vi "Test Executive.vi"(11 "Module Config":T30={"Name"="Test Executive", "Parent Q"=refnum, "Is Child?"=FALSE, "Index"=0, "Dirs"={"Root"=path "C:/MTE", "Config"=path "C:/MTE/Config", "Logs"=path "C:/MTE/Logs", "Reports"=path "C:/ATE/Reports", "App Data"=path "C:/ProgramData/Test Executive"}, "Simulate"=FALSE, "SimCtrl"=refnum}) -> ()   [LabVIEW 2018] (continued)
                          n1454 = control-ref of="Rigth Image"() -> (w3116:refnum<vi>)
                          n1455 = control-ref of="Left Image"() -> (w3115:refnum<vi>)
                          n1456 = call "Image.Load, Zoom and Center.vi"("Zoom Factor"=w3114, "2D Pict Ref"=w3116, "File"=w3125) -> ("error out"=w3117:errorcluster, "2D Pict"=→"Rigth Image":picture)  [unwired: 7 in]
                          n1457 = call "Image.Load, Zoom and Center.vi"("Zoom Factor"=w3114, "2D Pict Ref"=w3115, "File"=w3126) -> ("error out"=w3119:errorcluster, "2D Pict"=→"Left Image":picture)  [unwired: 7 in]
                          n1458 = Merge Errors(w3119, w3117) -> (w3118:errorcluster)
                          n1459 = case shown="Error" w3118 {
                            tunnel: w3122 -> [w3132 w3144]
                            tunnel: [w3132 w3143] -> w3121
                            tunnel: ["Wait for Input" "Result"] -> w3120
                            tunnel: w3117 -> [_ w3137]
                            tunnel: w3119 -> [_ w3138]
                            frame No Error {
                              n1460 = property on="OperNo 2" class="Bool"("DisabledEnum"=T36."Enabled" ("Disabled")) -> (error out=w3129:errorcluster)  [unwired: 2 in, 1 out]
                              n1461 = property on="OperOK 2" class="Bool"(error in=w3129, "DisabledEnum"=T36."Enabled" ("Disabled")) -> (error out=w3127:errorcluster)  [unwired: 1 in, 1 out]
                              n1462 = property on="OperOK 2" class="Bool"(error in=w3127, "Key Focus"=TRUE) -> ()  [unwired: 1 in, 2 out]
                            }
                            frame Error {
                              w3141 = T74 -5200 items=["No Error"=0, "Abort"=-2, "Misc"=-5000, "Fixture Error"=-5100, "File IO - General"=-5200, "FIle IO - Config Error"=-5201, "Instrument - General"=-5300, "Instrument - Serial Com"=-5301, "Instrument - Camera"=-5302, "Instrument - PS"=-5303, "Instrument - Oscilloscope"=-5304, "Instrument - Function Gen"=-5305, "Instrument - Load"=-5306, "Instrument - Meter"=-5307, "Instrument - Power Control"=-5308, "Instrument - Motion"=-5309, "Instrument - RF"=-5310, "System Exe"=-5400, "Image Processing"=-5500, "Communication"=-5600, "Script - Syntax Error"=-6000, "Script - Invalid Name or Param"=-6100, "Script - Timeout"=-6200, "Invalid Data"=-6300, "FW Update Error"=-6500] ("Std Code")
                              w3142 = T39 3 items=["LOG", "PASS", "FAIL", "ERROR"] ("Result.Status")
                              n1463 = case shown="Error" w3138 {
                                tunnel: w3137 -> [w3147 w3150]
                                tunnel: [w3146 w3149] -> w3135
                                frame No Error {
                                n1464 = case shown="Error" w3147 {
                                tunnel: [_ "Right image file load error."] -> w3146
                                frame No Error {
                                # "Will not get here"
                                }
                                frame Error {
                                }
                                }
                                }
                                frame Error {
                                n1465 = case shown="No Error" w3150 {
                                tunnel: ["Left image file load error." "Both left and right image file load error."] -> w3149
                                frame No Error {
                                }
                                frame Error {
                                }
                                }
                                }
                              }
                              n1466 = To Long Integer(number=w3141) -> (32bit integer=w3140:T74)
                              n1467 = Concatenate Strings("Image prompt error.  ", w3135) -> (w3136:string)
                              n1468 = Bundle By Name(cluster=w3144, "Result.Value"="Image Load Error", "Result.Status"=w3142, "Result.Code"=w3140, "Result.Desc"=w3136) -> (w3143:T80)
                            }
                          }
                        }
                        frame "Wait for Input" {
                          n1469 = while {
                            tunnel: w3155 -> [w3158]
                            tunnel: [w3157] -> w3154
                            tunnel: [w3156] -> w3153
                            stop <- w3159 stop-if-true
                            n1470 = event shown="[1] \"OperOK 2\", \"OperNo 2\": Value Change" {
                              selector: _ -> [_ _]
                              dyn-events: _ -> [_ _]
                              timeout: 100 -> [_ _]
                              tunnel: [w3163 TRUE] -> w3159
                              tunnel: w3158 -> [w3162 w3172]
                              tunnel: [w3162 w3171] -> w3157
                              tunnel: ["Done" "Result"] -> w3156
                              event Timeout {
                                n1471 = event-data() -> ()  [unwired: 1 in, 3 out]
                                n1472 = local read "Abort Flag"() -> (w3163:bool)
                              }
                              event "OperOK 2", "OperNo 2": Value Change {
                                n1473 = event-data() -> ()  [unwired: 1 in, 6 out]
                                n1474 = case shown="True" "OperOK 2" {
                                tunnel: ["Reject" "Accept"] -> w3169
                                tunnel: [w3176 w3179] -> w3168
                                tunnel: [5000 _] -> w3167
                                tunnel: ["Operator rejected image" _] -> w3166
                                tunnel: [_ TRUE] -> w3165
                                frame False {
                                w3176 = T39 2 items=["LOG", "PASS", "FAIL", "ERROR"] ("Result.Status")
                                }
                                frame True {
                                w3179 = T39 1 items=["LOG", "PASS", "FAIL", "ERROR"] ("Result.Status")
                                }
                                }
                                n1475 = Bundle By Name(cluster=w3172, "OK"=w3165, "Result.Value"=w3169, "Result.Status"=w3168, "Result.Code"=w3167, "Result.Desc"=w3166) -> (w3171:T80)
                              }
                            }
                          }
                        }
                        frame "Result" {
                          n1476 = Unbundle By Name(w3183) -> ("Result"=w3181:T43)
                          n1477 = Build Array(w3181) -> (w3186:T43[])
                          n1478 = To Variant(anything=w3186) -> (Variant=w3187:variant)
                          n1479 = call <vilib>:"Q.Enqueue Task.vi"("Top of Q"=TRUE, "Data1"=w3187, "Task Name"="Result - Attributes", "Q In"=w3184) -> ()  [unwired: 6 in, 2 out]
                        }
                        frame "Done", Default {
                          n1480 = Unbundle By Name(w3190) -> ("Opts.DispDetails"=w3193:bool)
                          n1481 = Select(t=1, s=w3193, f=0) -> (s? t:f=w3189:i32)
                          n1482 = local write "Test Status Tab"(w3189) -> ()
                          n1483 = local write "Test Status Tab Sel"(w3189) -> ()
                          n1484 = property on="OperNo 2" class="Bool"("DisabledEnum"=T36."Disabled and Grayed Out" ("Disabled")) -> ()  [unwired: 2 in, 2 out]
                          n1485 = property on="OperOK 2" class="Bool"("DisabledEnum"=T36."Disabled and Grayed Out" ("Disabled")) -> ()  [unwired: 2 in, 2 out]
                          n1486 = Unbundle By Name(w3195) -> ("OK"=w3194:bool)
                          n1487 = Select(t="Image Check: PASS" ("Category"), s=w3194, f="Image Check: FAIL" ("Category")) -> (s? t:f=w3200:string)
                          n1488 = property on="Status" class="Str"("Text.Text"=w3200, "Text.BGColor"=u32 13816530, "Blinking"=FALSE) -> ()  [unwired: 2 in, 2 out]
                        }
                      }
                    }
                  }
                  frame "PLCStart" {
                    n1489 = property on="PLC" class="Bool (strict)"() -> ("Visible"=w3206:bool)  [unwired: 2 in, 2 out]
                    n1490 = case shown="True" w3206 {
                      frame False {
                      }
                      frame True {
                        n1491 = call <vilib>:"Q.Enqueue Task.vi"("Q Name"="PLC", "Task Name"="TE PLC Start") -> ()  [unwired: 8 in, 2 out]
                      }
                    }
                  }
                  frame "Print_Label" {
                    # "Print_Label(Print_Text, URL)\n  If 2 arguements then will use this method.\n\nPrint_Label(Print_Text, File,CfgSection,CfgItem)\n  If 2 arguements then will use this method.\n  File can be full path or file name\n  If file name then folder is \"c:\\MTE\\[Test Station]\\Config\\\""
                    n1492 = Index Array(array=w3223) -> (element #1=w3219:string, element #2=w3221:string, element #3=w3220:string, element #4=w3222:string)  [unwired: 4 in]
                    n1493 = Unbundle By Name(w3212) -> ("Cfg.Dirs.Config"=w3211:path)
                    n1494 = Empty String/Path?(string/path=w3220) -> (empty?=w3218:bool)
                    n1495 = case shown="False" w3218 {
                      tunnel: w3222 -> [w3233 _]
                      tunnel: w3221 -> [w3232 w3240]
                      tunnel: w3220 -> [w3234 _]
                      tunnel: w3219 -> [w3235 w3241]
                      tunnel: [_ w3240] -> w3216
                      tunnel: [w3235 w3241] -> w3215
                      tunnel: [w3234 _] -> w3214
                      tunnel: [w3233 _] -> w3213
                      tunnel: w3211 -> [w3228 _]
                      tunnel: [w3225 _] -> w3210
                      frame False {
                        n1496 = String To Path(string=w3232) -> (path=w3226:path)
                        n1497 = Strip Path(path=w3226) -> (stripped path=w3230:path, name=w3227:string)
                        n1498 = Equal?(x=path "" ("stripped path"), y=w3230) -> (x = y?=w3229:bool)
                        n1499 = case shown="True" w3229 {
                          tunnel: w3228 -> [_ w3239]
                          tunnel: w3227 -> [_ w3238]
                          tunnel: w3226 -> [w3236 _]
                          tunnel: [w3236 w3237] -> w3225
                          frame False {
                          }
                          frame True {
                            n1500 = Build Path(base path=w3239, name or relative path=w3238) -> (appended path=w3237:path)
                          }
                        }
                      }
                      frame True {
                        # "Print_Label(URL,Print_Text)"
                      }
                    }
                    n1501 = call "TestExec.Print Label.vi"("CfgItem"=w3213, "URL"=w3216, "CfgSection"=w3214, "Text to Print"=w3215, "Config File"=w3210) -> ("error out"=w3217:errorcluster)  [unwired: 6 in]
                  }
                  frame "ProcessKill" {
                    # "ProcessKill(ProcessName)"
                    n1502 = Index Array(array=w3248) -> (element=w3247:string)  [unwired: 1 in]
                    n1503 = call "CmdExe.Get Processes with Kill Option.vi"("Kill Only 1 Instance"=TRUE, "Name Contains"=FALSE, "Kill Task"=TRUE, "Process Name"=w3247) -> ("Error Out"=w3242:errorcluster)  [unwired: 4 in, 3 out]
                    n1504 = call <vilib>:"Clear Errors.vi"("error in (no error)"=w3242) -> ()  [unwired: 5 in, 2 out]
                  }
                  frame "ProcessStatus" {
                    # "ProcessStatus(ProcessName, [RtnVarName])"
                    n1505 = Index Array(array=w3266) -> (element #1=w3265:string, element #2=w3252:string)  [unwired: 2 in]
                    n1506 = case shown="\"\"" w3252 {
                      selector: w3252 -> [w3267 _]
                      tunnel: [w3267 "ProcessIsRunning"] -> w3251
                      frame Default {
                      }
                      frame "" {
                      }
                    }
                    n1507 = call "CmdExe.Get Processes with Kill Option.vi"("Kill Only 1 Instance"=TRUE, "Name Contains"=FALSE, "Kill Task"=FALSE, "Process Name"=w3265) -> ("Error Out"=w3261:errorcluster, "Is Running"=w3249:bool)  [unwired: 4 in, 2 out]
                    n1508 = call <vilib>:"Clear Errors.vi"("error in (no error)"=w3261) -> ()  [unwired: 5 in, 2 out]
                    n1509 = Select(t="1", s=w3249, f="0") -> (s? t:f=w3254:string)
                    n1510 = Build Array(w3251, w3254) -> (w3253:string[])
                    n1511 = Unbundle By Name(w3257) -> ("SeqMgr"=w3260:refnum<class "SeqMgr.lvclass">)
                    n1512 = Build Array(w3253) -> (w3250:string[][])
                    n1513 = call <vilib>:"SeqMgr.Variables - Add, Replace.vi"("Name, Value"=w3250, "SeqMgr in"=w3260) -> ("SeqMgr out"=w3259:refnum<class "SeqMgr.lvclass">)  [unwired: 8 in, 1 out]
                    n1514 = Bundle By Name(cluster=w3257, "SeqMgr"=w3259) -> (w3258:T73)
                  }
                  frame "ReadINIConfig" {
                    # "ReadINIConfig(Folder,FileName,[Section1,Param1,Section2,Param2,...])\nReturns Vars: ConfigFileExists = 1 if exists, 0 otherwise\nFor each Section/Item pair  Sect1.Param1 = Value1\n                                                 Sect2.Param2 = Value2 . . ."
                    n1515 = while {
                      tunnel: w3270 -> [w3279]
                      shift-right: [w3282] -> w3271
                      shift-left: _ -> [w3283]
                      shift-right: [w3281] -> _
                      shift-left: "Init" -> [w3284]
                      tunnel: w3269 -> [w3278]
                      stop <- w3280 stop-if-true
                      n1516 = case shown="\"Init\"" w3284 {
                        tunnel: w3283 -> [_ w3304 w3314 w3340 w3375]
                        tunnel: [w3288 w3303 w3312 w3341 w3375] -> w3282
                        tunnel: ["File Exists" "Item List" w3313 "Done" _] -> w3281
                        tunnel: [_ _ _ _ TRUE] -> w3280
                        tunnel: w3279 -> [_ w3309 w3311 _ _]
                        tunnel: w3278 -> [_ w3300 _ _ _]
                        tunnel: [_ _ w3310 w3344 _] -> _
                        frame "Init" {
                          w3285 = FALSE  # Exists
                          w3286 = path ""  # Path
                          w3289 = string[][] []  # Items
                          w3290 = string[][] []  # Vars
                          n1517 = Bundle("Vars"=w3290, "Items"=w3289, "Path"=w3286, "Exists"=w3285) -> (w3288:T81)  [unwired: 1 in]
                        }
                        frame "File Exists" {
                          n1518 = Unbundle By Name(w3300) -> ("Cfg.Dirs.Config"=w3298:path)
                          n1519 = Index Array(array=w3309) -> (element #1=w3297:string, element #2=w3294:string)  [unwired: 2 in]
                          n1520 = Empty String/Path?(string/path=w3297) -> (empty?=w3299:bool)
                          n1521 = String To Path(string=w3297) -> (path=w3296:path)
                          n1522 = Select(t=w3298, s=w3299, f=w3296) -> (s? t:f=w3295:path)
                          n1523 = Build Path(base path=w3295, name or relative path=w3294) -> (appended path=w3293:path)
                          n1524 = call <vilib>:"File.Check if File or Folder Exists.vi"("Path"=w3293) -> ("Exists"=w3291:bool)  [unwired: 6 in, 4 out]
                          n1525 = Select(t="1", s=w3291, f="0") -> (s? t:f=w3307:string)
                          n1526 = Build Array("ConfigFileExists", w3307) -> (w3301:string[])
                          n1527 = Build Array(w3301) -> (w3302:string[][])
                          n1528 = Bundle By Name(cluster=w3304, "Path"=w3293, "Vars"=w3302, "Exists"=w3291) -> (w3303:T81)
                        }
                        frame "Item List" {
                          n1529 = Delete From Array(array=w3311, length=2, index=0) -> (array with subset deleted=w3315:string[])  [unwired: 1 out]
                          n1530 = Array Size(array=w3315) -> (size(s)=w3316:i32)
                          n1531 = case shown="Default" w3316 {
                            selector: w3316 -> [_ w3332]
                            tunnel: w3315 -> [_ w3331]
                            tunnel: w3314 -> [w3320 w3327]
                            tunnel: ["Done" "Get Items"] -> w3313
                            tunnel: [w3321 w3326] -> w3312
                            tunnel: [w3319 _] -> w3310
                            frame 0 {
                              n1532 = Unbundle By Name(w3320) -> ("Path"=w3323:path)
                              n1533 = call "File.Config, List Sections and Items in an INI File.vi"("Path"=w3323) -> ("error out"=w3319:errorcluster, "Items"=w3322:string[][])  [unwired: 9 in]
                              n1534 = Bundle By Name(cluster=w3320, "Items"=w3322) -> (w3321:T81)
                            }
                            frame Default {
                              n1535 = To Double Precision Float(number=w3332) -> (double precision float=w3334:dbl)
                              n1536 = Divide(x=w3334, y=2.0) -> (x/y=w3333:dbl)
                              n1537 = To Long Integer(number=w3333) -> (32bit integer=w3330:i32)
                              n1538 = Reshape Array(w3331, w3330, 2 ("dimension size")) -> (w3325:string[][])
                              n1539 = Bundle By Name(cluster=w3327, "Items"=w3325) -> (w3326:T81)
                            }
                          }
                        }
                        frame "Get Items" {
                          n1540 = Unbundle By Name(w3340) -> ("Items"=w3342:string[][], "Path"=w3343:path, "Exists"=w3336:bool)
                          n1541 = case shown="True" w3336 {
                            tunnel: [_ w3362] -> w3344
                            tunnel: w3343 -> [_ w3361]
                            tunnel: w3342 -> [w3347 w3356]
                            tunnel: [w3346 w3355] -> w3337
                            frame False {
                              # "Make empty Vars"
                              n1542 = for {
                                tunnel: w3347 -> [w3354] mode=indexing
                                tunnel: [w3349] -> w3346 mode=indexing
                                n1543 = Index Array(array=w3354) -> (element #1=w3353:string, element #2=w3352:string)  [unwired: 2 in]
                                n1544 = Concatenate Strings(w3353, ".", w3352) -> (w3351:string)
                                n1545 = Build Array(w3351, "") -> (w3349:string[])
                              }
                            }
                            frame True {
                              n1546 = call <vilib>:"Open Config Data.vi"("configuration file path"=w3361) -> ("error out"=w3359:errorcluster, "refnum"=w3360:T82)  [unwired: 8 in, 1 out]
                              n1547 = for {
                                tunnel: w3360 -> [w3374]
                                tunnel: [w3371] -> w3357
                                shift-right: [w3372] -> w3358
                                shift-left: w3359 -> [w3373]
                                tunnel: w3356 -> [w3370] mode=indexing
                                tunnel: [w3364] -> w3355 mode=indexing
                                tunnel: [w3363] -> _
                                n1548 = Index Array(array=w3370) -> (element #1=w3369:string, element #2=w3368:string)  [unwired: 2 in]
                                n1549 = call-poly <vilib>:"Read Key.vi"("section"=w3369, "error in (no error)"=w3373, "key"=w3368, "refnum"=w3374) -> ("error out"=w3372:errorcluster, "value"=w3366:string, "found?"=w3363:bool, "refnum out"=w3371:T82)  [unwired: 4 in]
                                n1550 = Concatenate Strings(w3369, ".", w3368) -> (w3367:string)
                                n1551 = Build Array(w3367, w3366) -> (w3364:string[])
                              }
                              n1552 = call <vilib>:"Close Config Data.vi"("error in (no error)"=w3358, "refnum"=w3357) -> ("error out"=w3362:errorcluster)  [unwired: 8 in, 1 out]
                            }
                          }
                          n1553 = Unbundle By Name(w3340) -> ("Vars"=w3339:string[][])
                          n1554 = Build Array (concatenate)(w3339, w3337) -> (w3338:string[][])
                          n1555 = Bundle By Name(cluster=w3340, "Vars"=w3338) -> (w3341:T81)
                        }
                        frame "Done", Default {
                        }
                      }
                    }
                    n1556 = Unbundle By Name(w3273) -> ("SeqMgr"=w3277:refnum<class "SeqMgr.lvclass">)
                    n1557 = Unbundle By Name(w3271) -> ("Vars"=w3275:string[][])
                    n1558 = call <vilib>:"SeqMgr.Variables - Add, Replace.vi"("Name, Value"=w3275, "SeqMgr in"=w3277) -> ("SeqMgr out"=w3276:refnum<class "SeqMgr.lvclass">)  [unwired: 8 in, 1 out]
                    n1559 = Bundle By Name(cluster=w3273, "SeqMgr"=w3276) -> (w3274:T73)
                  }
                  frame "RepeatMe" {
                    # "RepeatMe(WaitSecs)"
                    n1560 = Index Array(array=w3377) -> (element=w3385:string)  [unwired: 1 in]
                    n1561 = Fract/Exp String To Number(string=w3385) -> (number=w3384:dbl)  [unwired: 3 in, 1 out]
                    n1562 = Bundle By Name(cluster=w3380, "Repeat(s)"=w3384) -> (w3379:T73)
                    n1563 = Greater Or Equal To 0?(x=w3384) -> (x >= 0?=w3383:bool)
                    n1564 = case shown="False" w3383 {
                      tunnel: ["Repeat Sequence turned OFF." w3391] -> w3381
                      tunnel: w3384 -> [_ w3389]
                      frame False {
                      }
                      frame True {
                        n1565 = Number To Fractional String(number=w3389, precision (6)=i16 1) -> (F-format string=w3387:string)  [unwired: 2 in]
                        n1566 = Format Into String(format string="Repeat Sequence turned ON, set for %s secs.", w3387) -> (resulting string=w3391:string)  [unwired: 2 in, 1 out]
                      }
                    }
                    n1567 = Unbundle By Name(w3378) -> ("Log"=w3382:refnum<class "Event Notification.lvclass">)
                    n1568 = call <vilib>:"Event Notification.Status Message.vi"("Message"=w3381, "Event Notification in"=w3382) -> ()  [unwired: 10 in]
                  }
                  frame "RunUtility" {
                    w3393 = TRUE ("Top of Q")
                    n1569 = Index Array(array=w3417) -> (element=w3420:string)  [unwired: 1 in]
                    n1570 = Unbundle By Name(w3416) -> ("Cfg.Dirs.Config"=w3422:path)
                    n1571 = Unbundle By Name(w3394) -> ("UUT Dir"=w3414:path, "TimeOut(s)"=w3415:dbl)
                    n1572 = Unbundle By Name(w3394) -> ("SeqMgr"=w3419:refnum<class "SeqMgr.lvclass">)
                    n1573 = Build Path(base path=w3422, name or relative path=w3420) -> (appended path=w3421:path)
                    n1574 = call <vilib>:"SeqMgr.Variables - Get.vi"("SeqMgr in"=w3419) -> ("Vars"=w3418:variant)  [unwired: 8 in, 2 out]
                    n1575 = call "TestExec.Run Executable and Parse Results V2vi.vi"("Vars"=w3418, "Timeout(s)"=w3415, "Output Folder"=w3414, "Utility Config File"=w3421) -> ("Error"=w3392:errorcluster, "RTN Data"=w3412:T83)  [unwired: 6 in]
                    n1576 = Unbundle By Name(w3412) -> ("Vars"=w3405:string[][], "SW Items"=w3404:T31[], "FileObjs"=w3402:T29[], "MeasData"=w3403:T38[])
                    n1577 = call <vilib>:"Clear Errors.vi"("error in (no error)"=w3392) -> ()  [unwired: 5 in, 2 out]
                    n1578 = To Variant(anything=w3404) -> (Variant=w3397:variant)
                    n1579 = To Variant(anything=w3402) -> (Variant=w3398:variant)
                    n1580 = To Variant(anything=w3403) -> (Variant=w3399:variant)
                    n1581 = call <vilib>:"Q.Enqueue Task.vi"("Top of Q"=w3393, "Data1"=w3399, "Task Name"="Result - Measurements", "Q In"=w3411) -> ("Q Out"=w3400:refnum<queue>)  [unwired: 6 in, 1 out]
                    n1582 = local read "Variables"() -> (w3409:string[][])
                    n1583 = Unbundle By Name(w3394) -> ("SeqMgr"=w3407:refnum<class "SeqMgr.lvclass">)
                    n1584 = call <vilib>:"Q.Enqueue Task.vi"("Top of Q"=w3393, "Data1"=w3398, "Task Name"="Result - File Objs" ("Cmd"), "Q In"=w3400) -> ("Q Out"=w3401:refnum<queue>)  [unwired: 6 in, 1 out]
                    n1585 = call <vilib>:"Q.Enqueue Task.vi"("Top of Q"=w3393, "Data1"=w3397, "Task Name"="Client - SW Items", "Q In"=w3401) -> ()  [unwired: 6 in, 2 out]
                    n1586 = call "TestExec.Add New 1D Items to 2D List, Overwrite if is existing.vi"("New Items"=w3405, "Item List"=w3409) -> ("Item List Out"=w3410:string[][])  [unwired: 9 in]
                    n1587 = call <vilib>:"SeqMgr.Variables - Add, Replace.vi"("Name, Value"=w3405, "SeqMgr in"=w3407) -> ("SeqMgr out"=w3408:refnum<class "SeqMgr.lvclass">)  [unwired: 8 in, 1 out]
                    n1588 = Bundle By Name(cluster=w3394, "SeqMgr"=w3408) -> (w3406:T73)
                    n1589 = local write "Variables"(w3410) -> ()
                  }
                  frame "RunExe" {
                    n1590 = Unbundle By Name(w3435) -> ("UUT Dir"=w3430:path, "TimeOut(s)"=w3439:dbl)
                    n1591 = Delete From Array(array=w3429, length=1, index=0) -> (deleted portion=w3423:string[], array with subset deleted=w3425:string[])
                    n1592 = Unbundle By Name(w3435) -> ("SeqMgr"=w3441:refnum<class "SeqMgr.lvclass">)
                    n1593 = Index Array(array=w3423) -> (element=w3424:string)  [unwired: 1 in]
                    n1594 = local write "Args"(w3425) -> ()
                    n1595 = call <vilib>:"SeqMgr.Variables - Get.vi"("SeqMgr in"=w3441) -> ("Vars"=w3440:variant)  [unwired: 8 in, 2 out]
                    n1596 = String To Path(string=w3424) -> (path=w3426:path)
                    n1597 = local write "Exe Path"(w3426) -> ()
                    n1598 = call "TestExec.Run Executable and Rtn.vi"("Vars"=w3440, "Timeout(s)"=w3439, "Log Dir"=w3430, "Input"=w3429) -> ("Error"=w3431:errorcluster, "RTN Data"=w3434:T83)  [unwired: 6 in]
                    n1599 = call <vilib>:"Clear Errors.vi"("error in (no error)"=w3431) -> ()  [unwired: 5 in, 2 out]
                    n1600 = Unbundle By Name(w3434) -> ("MeasData"=w3433:T38[])
                    n1601 = To Variant(anything=w3433) -> (Variant=w3436:variant)
                    n1602 = call <vilib>:"Q.Enqueue Task.vi"("Top of Q"=TRUE, "Data1"=w3436, "Task Name"="Result - Measurements", "Q In"=w3437) -> ()  [unwired: 6 in, 2 out]
                  }
                  frame "SectionStart" {
                    # "SectionStart(Name)"
                    n1603 = Unbundle By Name(w3446) -> ("SectCtr"=w3466:T72, "Data.Meas"=w3463:T38[])
                    n1604 = Index Array(array=w3442) -> (element=w3459:string)  [unwired: 1 in]
                    n1605 = To Upper Case(1:w3459) -> (0:w3452:string)
                    n1606 = call <vilib>:"Q.Enqueue Task.vi"("Top of Q"=TRUE, "Task Name"="Update Result Table", "Q In"=w3443) -> ()  [unwired: 7 in, 2 out]
                    n1607 = call "Step Counter.Step Count Controller.vi"("Step Action"=Step_Counter.Action."Section Start", "Step State"=w3466) -> ("Step"=w3461:string, "Step State Out"=w3465:T72, "Cntr"=w3454:i32)  [unwired: 7 in]
                    n1608 = Bundle By Name(cluster=T38 {"Cnt"=0, "Step"="", "Category"="", "Name"="", "Value"="", "Units"="", "LimType"="", "LL"="", "UL"="", "Status"=0, "Code"=0, "Desc"="", "Time"=timestamp(0 s since 1904-01-01)} ("Meas"), "Step"=w3461, "Cnt"=w3454, "Category"="Heading", "Name"=w3452, "Value"="==================") -> (w3458:T38)
                    n1609 = Build Array (concatenate)(w3463, w3458) -> (w3462:T38[])
                    n1610 = Bundle By Name(cluster=w3446, "SectCtr"=w3465, "Data.Meas"=w3462) -> (w3445:T73)
                    n1611 = Unbundle By Name(w3444) -> ("Log"=w3451:refnum<class "Event Notification.lvclass">)
                    n1612 = Format Into String(format string="Section Start: %s", w3452) -> (resulting string=w3450:string)  [unwired: 2 in, 1 out]
                    n1613 = call <vilib>:"Event Notification.Status Message.vi"("Log"=TRUE, "Level"=Event_Log.Log_Level."Verbose", "Message"=w3450, "Event Notification in"=w3451) -> ()  [unwired: 8 in]
                  }
                  frame "SendDataToSta" {
                    n1614 = Unbundle By Name(w3469) -> ("ResultState"=w3473:T63, "Data.Meas"=w3468:T38[], "StaApp"=w3467:string)
                    n1615 = To Variant(anything=w3468) -> (Variant=w3470:variant)
                    n1616 = call <vilib>:"Q.Enqueue Task.vi"("Top of Q"=TRUE, "Data1"=w3470, "Q Name"=w3467, "Task Name"="Test Meas Data") -> ()  [unwired: 6 in, 2 out]
                    n1617 = To Variant(anything=w3473) -> (Variant=w3474:variant)
                    n1618 = call <vilib>:"Q.Enqueue Task.vi"("Top of Q"=TRUE, "Data1"=w3474, "Q Name"=w3467, "Task Name"="Test Status") -> ()  [unwired: 6 in, 2 out]
                  }
                  frame "SequenceConfig" {
                    # "If name exists, over write.\nElse append."
                    # "SequenceConfig(Name, Value)"
                    n1619 = Unbundle By Name(w3479) -> ("RptHdr.Test Sequence"=w3489:T49)
                    n1620 = Unbundle By Name(w3489) -> ("Config.Config_Item"=w3486:cluster{"Name":string, "Value":string}[])
                    n1621 = for {
                      tunnel: w3486 -> [w3498] mode=indexing
                      tunnel: [w3497] -> w3485 mode=indexing
                      n1622 = Unbundle By Name(w3498) -> ("Name"=w3497:string)
                    }
                    n1623 = Index Array(array=w3477) -> (element #1=w3480:string, element #2=w3483:string)  [unwired: 2 in]
                    n1624 = Bundle By Name(cluster=cluster{"Name":string, "Value":string} {"Name"="", "Value"=""} ("Setup"), "Name"=w3480, "Value"=w3483) -> (w3482:cluster{"Name":string, "Value":string})
                    n1625 = Search 1D Array(1D array=w3485, element=w3480) -> (index of element=w3481:i32)  [unwired: 1 in]
                    n1626 = case shown="0, Default" w3481 {
                      selector: w3481 -> [w3490 _]
                      tunnel: w3486 -> [w3493 w3496]
                      tunnel: [w3492 w3495] -> w3488
                      tunnel: w3482 -> [w3491 w3494]
                      frame 0, Default {
                        n1627 = Replace Array Subset(array=w3493, new element=w3491, index=w3490) -> (w3492:cluster{"Name":string, "Value":string}[])
                      }
                      frame -1 {
                        n1628 = Build Array (concatenate)(w3496, w3494) -> (w3495:cluster{"Name":string, "Value":string}[])
                      }
                    }
                    n1629 = Bundle By Name(cluster=w3489, "Config.Config_Item"=w3488) -> (w3487:T49)
                    n1630 = Bundle By Name(cluster=w3479, "RptHdr.Test Sequence"=w3487) -> (w3478:T73)
                  }
                  frame "SetDisableResults" {
                    # "SetDisableResults(Enabled)\n1 = Enabled, 0 = Disabled"
                    n1631 = Index Array(array=w3499) -> (element=w3512:string)  [unwired: 1 in]
                    n1632 = Unbundle By Name(w3500) -> ("Opts.DisResults"=w3507:bool)
                    n1633 = Equal?(x=w3512, y="1") -> (x = y?=w3509:bool)
                    n1634 = Or(x=w3507, y=w3509) -> (x .or. y?=w3508:bool)
                    n1635 = Select(t="ON", s=w3509, f="OFF") -> (s? t:f=w3510:string)
                    n1636 = Bundle By Name(cluster=w3500, "DisableResults"=w3508) -> (w3502:T73)
                    n1637 = Unbundle By Name(w3501) -> ("Log"=w3506:refnum<class "Event Notification.lvclass">)
                    n1638 = Format Into String(format string="Set Disable Results to %s.", w3510) -> (resulting string=w3505:string)  [unwired: 2 in, 1 out]
                    n1639 = call <vilib>:"Event Notification.Status Message.vi"("Log"=TRUE, "Level"=Event_Log.Log_Level."Verbose", "Message"=w3505, "Event Notification in"=w3506) -> ()  [unwired: 8 in]
                  }
                  frame "SetSN" {
                    n1640 = Index Array(array=w3535) -> (element=w3525:string)  [unwired: 1 in]
                    n1641 = Unbundle By Name(w3522) -> ("Opts.SNRouteCk"=w3521:bool, "Opts.NotValSN"=w3527:bool, "Lists.UUTRoutes"=w3520:string[])
                    n1642 = Unbundle By Name(w3522) -> ("StaApp"=w3533:string)
                    n1643 = Bundle By Name(cluster=w3522, "RptUUT.UUTInfo.SN"=w3525) -> (w3518:T73)
                    n1644 = To Variant(anything=w3525) -> (Variant=w3531:variant)
                    n1645 = local write "SN"(w3525) -> ()
                    n1646 = local write "SN Rslt"(w3525) -> ()
                    n1647 = call <vilib>:"Q.Enqueue Task.vi"("Data1"=w3531, "Q Name"=w3533, "Task Name"="Update SN") -> ()  [unwired: 7 in, 2 out]
                    n1648 = Format Into String(format string="Sequence reassigned SN to %s" ("Message"), w3525) -> (resulting string=w3538:string)  [unwired: 2 in, 1 out]
                    n1649 = Build Array("SN", w3525) -> (w3524:string[])
                    n1650 = Unbundle By Name(w3526) -> ("Log"=w3539:refnum<class "Event Notification.lvclass">)
                    n1651 = Build Array(w3524) -> (w3523:string[][])
                    n1652 = case shown="True" w3527 {
                      tunnel: [w3550 _] -> _
                      tunnel: w3525 -> [w3549 _]
                      tunnel: w3523 -> [w3548 w3566]
                      tunnel: [w3546 w3566] -> w3516
                      tunnel: [w3543 w3565] -> w3517
                      tunnel: w3521 -> [w3542 _]
                      tunnel: w3520 -> [w3541 _]
                      tunnel: w3518 -> [w3540 w3565]
                      frame False {
                        n1653 = control-ref of="SN"() -> (w3551:refnum<vi>)
                        n1654 = call "TestExec.SN Valid and Route Check.vi"("Process Steps"=w3541, "SN Indicator"=w3551, "SN"=w3549, "Route Check"=w3542) -> ("Message"=w3544:string, "Status"=w3545:bool, "error IO"=w3550:errorcluster)  [unwired: 4 in, 1 out]
                        n1655 = case shown="True" w3545 {
                          tunnel: w3548 -> [w3560 w3564]
                          tunnel: string[][] [["Error", "1"]] ("appended array") -> [w3559 _]
                          tunnel: [w3558 w3564] -> w3546
                          tunnel: w3540 -> [w3555 w3562]
                          tunnel: [w3556 w3561] -> w3543
                          tunnel: w3544 -> [w3553 _]
                          frame False {
                            n1656 = Build Array (concatenate)(w3560, w3559) -> (w3558:string[][])
                            n1657 = local write "UUT SN Status"(w3553) -> ()
                            n1658 = Bundle By Name(cluster=w3555, "PreTestCk.SNErr"=TRUE, "ResultState.State"=SeqMgr.Result_State_Enum."ERROR" ("State"), "ResultState.Code"=-8002, "ResultState.Description"=w3553) -> (w3556:T73)
                          }
                          frame True {
                            # "SN is OK"
                            n1659 = Bundle By Name(cluster=w3562, "PreTestCk.SNErr"=FALSE) -> (w3561:T73)
                          }
                        }
                      }
                      frame True {
                      }
                    }
                    n1660 = call <vilib>:"Event Notification.Status Message.vi"("Display"=TRUE ("Log"), "Level"=Event_Log.Log_Level."Verbose", "Message"=w3538, "Event Notification in"=w3539) -> ()  [unwired: 8 in]
                    n1661 = Unbundle By Name(w3517) -> ("SeqMgr"=w3530:refnum<class "SeqMgr.lvclass">)
                    n1662 = call <vilib>:"SeqMgr.Variables - Add, Replace.vi"("Name, Value"=w3516, "SeqMgr in"=w3530) -> ("SeqMgr out"=w3529:refnum<class "SeqMgr.lvclass">)  [unwired: 8 in, 1 out]
                    n1663 = Bundle By Name(cluster=w3517, "SeqMgr"=w3529) -> (w3519:T73)
                  }
                  frame "SetTimeout" {
                    n1664 = Index Array(array=w3570) -> (element=w3581:string)  [unwired: 1 in]
                    n1665 = Fract/Exp String To Number(string=w3581) -> (number=w3580:dbl)  [unwired: 3 in, 1 out]
                    n1666 = In Range and Coerce(upper limit=1000.0, x=w3580, lower limit=1.0) -> (coerced(x)=w3578:dbl)  [unwired: 1 out]
                    n1667 = call <vilib>:"Q.Enqueue Task.vi"("Top of Q"=TRUE, "Task Name"="Sta Set TimeOut", "Q In"=w3568) -> ()  [unwired: 7 in, 2 out]
                    n1668 = Bundle By Name(cluster=w3572, "TimeOut(s)"=w3578) -> (w3571:T73)
                    n1669 = Unbundle By Name(w3573) -> ("Log"=w3577:refnum<class "Event Notification.lvclass">)
                    n1670 = Format Into String(format string="Function call timeout set to %.2f secs.", w3578) -> (resulting string=w3576:string)  [unwired: 2 in, 1 out]
                    n1671 = call <vilib>:"Event Notification.Status Message.vi"("Log"=TRUE, "Level"=Event_Log.Log_Level."Verbose", "Message"=w3576, "Event Notification in"=w3577) -> ()  [unwired: 8 in]
                  }
                  frame "GetTimeSecs" {
                    n1672 = Index Array(array=w3588) -> (element=w3585:string)  [unwired: 1 in]
                    n1673 = call <vilib>:"High Resolution Relative Seconds.vi"() -> ("relative seconds"=w3587:dbl)
                    n1674 = Number To Fractional String(number=w3587) -> (F-format string=w3586:string)  [unwired: 3 in]
                    n1675 = Build Array(w3585, w3586) -> (w3584:string[])
                    n1676 = Unbundle By Name(w3590) -> ("SeqMgr"=w3593:refnum<class "SeqMgr.lvclass">)
                    n1677 = Build Array(w3584) -> (w3591:string[][])
                    n1678 = call <vilib>:"SeqMgr.Variables - Add, Replace.vi"("Name, Value"=w3591, "SeqMgr in"=w3593) -> ("SeqMgr out"=w3592:refnum<class "SeqMgr.lvclass">)  [unwired: 8 in, 1 out]
                    n1679 = Bundle By Name(cluster=w3590, "SeqMgr"=w3592) -> (w3589:T73)
                  }
                  frame "GetDurationSecs" {
                    n1680 = Index Array(array=w3601) -> (element #1=w3599:string, element #2=w3597:string)  [unwired: 2 in]
                    n1681 = Fract/Exp String To Number(string=w3597) -> (number=w3595:dbl)  [unwired: 3 in, 1 out]
                    n1682 = call <vilib>:"High Resolution Relative Seconds.vi"() -> ("relative seconds"=w3596:dbl)
                    n1683 = Subtract(x=w3596, y=w3595) -> (x-y=w3594:dbl)
                    n1684 = Number To Fractional String(number=w3594) -> (F-format string=w3600:string)  [unwired: 3 in]
                    n1685 = Build Array(w3599, w3600) -> (w3598:string[])
                    n1686 = Unbundle By Name(w3603) -> ("SeqMgr"=w3606:refnum<class "SeqMgr.lvclass">)
                    n1687 = Build Array(w3598) -> (w3604:string[][])
                    n1688 = call <vilib>:"SeqMgr.Variables - Add, Replace.vi"("Name, Value"=w3604, "SeqMgr in"=w3606) -> ("SeqMgr out"=w3605:refnum<class "SeqMgr.lvclass">)  [unwired: 8 in, 1 out]
                    n1689 = Bundle By Name(cluster=w3603, "SeqMgr"=w3605) -> (w3602:T73)
                  }
                  frame "SetVar", "SetVariable" {
                    # "SetVariable(Name,Value)"
                    n1690 = Unbundle By Name(w3609) -> ("SeqMgr"=w3620:refnum<class "SeqMgr.lvclass">)
                    n1691 = Index Array(array=w3607) -> (element #1=w3616:string, element #2=w3615:string)  [unwired: 2 in]
                    n1692 = Build Array(w3607) -> (w3618:string[][])
                    n1693 = call <vilib>:"SeqMgr.Variables - Add, Replace.vi"("Name, Value"=w3618, "SeqMgr in"=w3620) -> ("SeqMgr out"=w3619:refnum<class "SeqMgr.lvclass">)  [unwired: 8 in, 1 out]
                    n1694 = Bundle By Name(cluster=w3609, "SeqMgr"=w3619) -> (w3608:T73)
                    n1695 = Format Into String(format string="Set Var, %s, %s", w3616, w3615) -> (resulting string=w3613:string)  [unwired: 2 in, 1 out]
                    n1696 = Unbundle By Name(w3610) -> ("Log"=w3614:refnum<class "Event Notification.lvclass">)
                    n1697 = call <vilib>:"Event Notification.Status Message.vi"("Log"=TRUE, "Level"=Event_Log.Log_Level."Debug0", "Message"=w3613, "Event Notification in"=w3614) -> ()  [unwired: 8 in]
                  }
                  frame "SubSectionEnd" {
                    # "SubSectionEnd()"
                    n1698 = Unbundle By Name(w3622) -> ("SectCtr"=w3625:T72)
                    n1699 = call "Step Counter.Step Count Controller.vi"("Step Action"=Step_Counter.Action."Sub Section End", "Step State"=w3625) -> ("Step State Out"=w3624:T72)  [unwired: 7 in, 2 out]
                    n1700 = Bundle By Name(cluster=w3622, "SectCtr"=w3624) -> (w3621:T73)
                  }
                  frame "SubSectionStart" {
                    # "SubSectionStart(Name)"
                    n1701 = Index Array(array=w3629) -> (element=w3642:string)  [unwired: 1 in]
                    n1702 = To Upper Case(1:w3642) -> (0:w3639:string)
                    n1703 = Unbundle By Name(w3628) -> ("SectCtr"=w3647:T72, "Data.Meas"=w3645:T38[])
                    n1704 = call <vilib>:"Q.Enqueue Task.vi"("Top of Q"=TRUE, "Task Name"="Update Result Table", "Q In"=w3648) -> ()  [unwired: 7 in, 2 out]
                    n1705 = call "Step Counter.Step Count Controller.vi"("Step Action"=Step_Counter.Action."Sub Section Start", "Step State"=w3647) -> ("Step"=w3643:string, "Step State Out"=w3646:T72, "Cntr"=w3640:i32)  [unwired: 7 in]
                    n1706 = Bundle By Name(cluster=T38 {"Cnt"=0, "Step"="", "Category"="", "Name"="", "Value"="", "Units"="", "LimType"="", "LL"="", "UL"="", "Status"=0, "Code"=0, "Desc"="", "Time"=timestamp(0 s since 1904-01-01)} ("Meas"), "Step"=w3643, "Cnt"=w3640, "Category"="Heading", "Name"=w3639, "Value"="- - - - - - - - - -" ("Category")) -> (w3641:T38)
                    n1707 = Build Array (concatenate)(w3645, w3641) -> (w3644:T38[])
                    n1708 = Bundle By Name(cluster=w3628, "SectCtr"=w3646, "Data.Meas"=w3644) -> (w3626:T73)
                    n1709 = Unbundle By Name(w3627) -> ("Log"=w3638:refnum<class "Event Notification.lvclass">)
                    n1710 = Format Into String(format string="SubSection Start: %s", w3639) -> (resulting string=w3637:string)  [unwired: 2 in, 1 out]
                    n1711 = call <vilib>:"Event Notification.Status Message.vi"("Log"=TRUE, "Level"=Event_Log.Log_Level."Verbose", "Message"=w3637, "Event Notification in"=w3638) -> ()  [unwired: 8 in]
                  }
                  frame "TimeLog" {
                    n1712 = Index Array(array=w3652) -> (element=w3655:string)  [unwired: 1 in]
                    n1713 = Unbundle By Name(w3653) -> ("Log"=w3656:refnum<class "Event Notification.lvclass">)
                    n1714 = call <vilib>:"Event Notification.Status Message.vi"("Display"=TRUE, "Log"=TRUE, "Level"=Event_Log.Log_Level."Normal", "Message"=w3655, "Event Notification in"=w3656) -> ()  [unwired: 7 in]
                  }
                  frame "XlinkPartInitReport" {
                    # "XlinkPartInitReport(DestinationFolder,Batch,Name)"
                    n1715 = Unbundle By Name(w3660) -> ("RptHdr.Test Run.Start Time"=w3668:timestamp, "RptUUT.UUTInfo.SN"=w3667:string, "RptHdr.Test Run.Operator"=w3666:string)
                    n1716 = Index Array(array=w3659) -> (element #1=w3663:string, element #2=w3662:string, element #3=w3661:string)  [unwired: 3 in]
                    n1717 = String To Path(string=w3663) -> (path=w3664:path)
                    n1718 = call "Result.Generate Xlink PN Init Report XML.vi"("Name"=w3661, "Batch"=w3662, "Time Offset"=-1.0, "Folder"=w3664, "Operator"=w3666, "SN"=w3667, "StartTime"=w3668) -> ()  [unwired: 3 in, 2 out]
                  }
                  frame Default {
                    w3672 = T74 -6100 items=["No Error"=0, "Abort"=-2, "Misc"=-5000, "Fixture Error"=-5100, "File IO - General"=-5200, "FIle IO - Config Error"=-5201, "Instrument - General"=-5300, "Instrument - Serial Com"=-5301, "Instrument - Camera"=-5302, "Instrument - PS"=-5303, "Instrument - Oscilloscope"=-5304, "Instrument - Function Gen"=-5305, "Instrument - Load"=-5306, "Instrument - Meter"=-5307, "Instrument - Power Control"=-5308, "Instrument - Motion"=-5309, "Instrument - RF"=-5310, "System Exe"=-5400, "Image Processing"=-5500, "Communication"=-5600, "Script - Syntax Error"=-6000, "Script - Invalid Name or Param"=-6100, "Script - Timeout"=-6200, "Invalid Data"=-6300, "FW Update Error"=-6500] ("Std Code")
                    n1719 = Format Into String(format string="Invalid sequence function name: \"%s\".", w3670) -> (resulting string=w3673:string)  [unwired: 2 in, 1 out]
                    n1720 = call "Error.Set-Change Error Info.vi"("Std Code"=w3672, "Description"=w3673, "Set Error"=TRUE) -> ("error out"=w3669:errorcluster)  [unwired: 8 in]
                  }
                }
              }
              frame Error {
                w3681 = T74 -6000 items=["No Error"=0, "Abort"=-2, "Misc"=-5000, "Fixture Error"=-5100, "File IO - General"=-5200, "FIle IO - Config Error"=-5201, "Instrument - General"=-5300, "Instrument - Serial Com"=-5301, "Instrument - Camera"=-5302, "Instrument - PS"=-5303, "Instrument - Oscilloscope"=-5304, "Instrument - Function Gen"=-5305, "Instrument - Load"=-5306, "Instrument - Meter"=-5307, "Instrument - Power Control"=-5308, "Instrument - Motion"=-5309, "Instrument - RF"=-5310, "System Exe"=-5400, "Image Processing"=-5500, "Communication"=-5600, "Script - Syntax Error"=-6000, "Script - Invalid Name or Param"=-6100, "Script - Timeout"=-6200, "Invalid Data"=-6300, "FW Update Error"=-6500] ("Std Code")
                n1721 = call <vilib>:"Space Constant.vi"() -> ("String"=w3678:string)
                n1722 = Concatenate Strings(w3680, w3678, w3679) -> (w3677:string)
                n1723 = Format Into String(format string="Invalid Data to task %s. Expected 1D string.", w3677) -> (resulting string=w3682:string)  [unwired: 2 in, 1 out]
                n1724 = call "Error.Set-Change Error Info.vi"("Std Code"=w3681, "Description"=w3682) -> ("error out"=w3676:errorcluster)  [unwired: 9 in]
              }
            }
          }
          frame "Set Comment" {
            # "Set SN(SN)"
            n1725 = Variant To Data(type="", Variant=w3697) -> (data=w3686:string)  [unwired: 1 in, 1 out]
            n1726 = Bundle By Name(cluster=w3696, "RptHdr.Test Run.Comment"=w3686) -> (w3693:T73)
            n1727 = local write "Comment"(w3686) -> ()
            n1728 = String Length(string=w3686) -> (length=w3687:i32)
            n1729 = case shown="0..18" w3687 {
              tunnel: [u32 16 ("F2") u32 20 ("F1")] -> w3685
              frame Default {
              }
              frame 0..18 {
              }
            }
            n1730 = Format Into String(format string="Automation reassigned Comment to %s" ("Message"), w3686) -> (resulting string=w3688:string)  [unwired: 2 in, 1 out]
            n1731 = Unbundle By Name(w3689) -> ("Log"=w3692:refnum<class "Event Notification.lvclass">)
            n1732 = property on="SN" class="Str"("Text.FontSize"=w3685) -> ()  [unwired: 2 in, 2 out]
            n1733 = call <vilib>:"Event Notification.Status Message.vi"("Log"=TRUE, "Level"=Event_Log.Log_Level."Verbose", "Message"=w3688, "Event Notification in"=w3692) -> ()  [unwired: 8 in]
          }
          frame "Set Sequence" {
            # "Set Position(Int)"
            n1734 = Variant To Data(type="", Variant=w3714) -> (data=w3701:string)  [unwired: 1 in, 1 out]
            n1735 = property on="Sequence" class="Ring (strict)"() -> ("Strings []"=w3706:string[])  [unwired: 2 in, 2 out]
            n1736 = To Lower Case(string=w3701) -> (all lower case string=w3704:string)
            n1737 = To Lower Case(string=w3706) -> (all lower case string=w3705:string[])
            n1738 = Search 1D Array(1D array=w3705, element=w3704) -> (index of element=w3702:i32)  [unwired: 1 in]
            n1739 = case shown="0, Default" w3702 {
              selector: w3702 -> [_ w3721]
              tunnel: w3701 -> [w3716 _]
              tunnel: [w3715 _] -> w3700
              frame -1 {
                w3719 = T74 -6100 items=["No Error"=0, "Abort"=-2, "Misc"=-5000, "Fixture Error"=-5100, "File IO - General"=-5200, "FIle IO - Config Error"=-5201, "Instrument - General"=-5300, "Instrument - Serial Com"=-5301, "Instrument - Camera"=-5302, "Instrument - PS"=-5303, "Instrument - Oscilloscope"=-5304, "Instrument - Function Gen"=-5305, "Instrument - Load"=-5306, "Instrument - Meter"=-5307, "Instrument - Power Control"=-5308, "Instrument - Motion"=-5309, "Instrument - RF"=-5310, "System Exe"=-5400, "Image Processing"=-5500, "Communication"=-5600, "Script - Syntax Error"=-6000, "Script - Invalid Name or Param"=-6100, "Script - Timeout"=-6200, "Invalid Data"=-6300] ("Std Code")
                n1740 = Format Into String(format string="Error attempted to set to nonexistant sequence: \"%s\"." ("Description"), w3716) -> (resulting string=w3717:string)  [unwired: 2 in, 1 out]
                n1741 = call "Error.Set-Change Error Info.vi"("Std Code"=w3719, "Description"=w3717, "Set Error"=TRUE) -> ("error out"=w3715:errorcluster)  [unwired: 8 in]
              }
              frame 0, Default {
                n1742 = To Unsigned Word Integer(number=w3721) -> (unsigned 16bit integer=w3722:u16)
                n1743 = property on="Sequence" class="Ring (strict)"("Value"=w3722) -> ()  [unwired: 2 in, 2 out]
              }
            }
            n1744 = Unbundle By Name(w3711) -> ("Log"=w3710:refnum<class "Event Notification.lvclass">)
            n1745 = Format Into String(format string="Set Sequence to %s" ("Message"), w3701) -> (resulting string=w3703:string)  [unwired: 2 in, 1 out]
            n1746 = call <vilib>:"Event Notification.Status Message.vi"("Log"=TRUE, "Level"=Event_Log.Log_Level."Normal", "Message"=w3703, "Event Notification in"=w3710) -> ()  [unwired: 8 in]
          }
          frame "Set SN" {
            # "Set SN(SN)"
            n1747 = Variant To Data(type="", Variant=w3739) -> (data=w3725:string)  [unwired: 1 in, 1 out]
            n1748 = Bundle By Name(cluster=w3738, "RptUUT.UUTInfo.SN"=w3725) -> (w3724:T73)
            n1749 = local write "SN"(w3725) -> ()
            n1750 = local write "SN Rslt"(w3725) -> ()
            n1751 = Build Array("SN", w3725) -> (w3726:string[])
            n1752 = Unbundle By Name(w3724) -> ("SeqMgr"=w3730:refnum<class "SeqMgr.lvclass">)
            n1753 = Build Array(w3726) -> (w3728:string[][])
            n1754 = call <vilib>:"SeqMgr.Variables - Add, Replace.vi"("Name, Value"=w3728, "SeqMgr in"=w3730) -> ("SeqMgr out"=w3729:refnum<class "SeqMgr.lvclass">)  [unwired: 8 in, 1 out]
            n1755 = Bundle By Name(cluster=w3724, "SeqMgr"=w3729) -> (w3723:T73)
            n1756 = Format Into String(format string="Automation reassigned SN to %s" ("Message"), w3725) -> (resulting string=w3731:string)  [unwired: 2 in, 1 out]
            n1757 = Unbundle By Name(w3732) -> ("Log"=w3735:refnum<class "Event Notification.lvclass">)
            n1758 = call <vilib>:"Event Notification.Status Message.vi"("Log"=TRUE, "Level"=Event_Log.Log_Level."Verbose", "Message"=w3731, "Event Notification in"=w3735) -> ()  [unwired: 8 in]
          }
          frame "Set UUT Pos" {
            # "Set Position(Int)"
            n1759 = Variant To Data(type="", Variant=w3751) -> (data=w3741:string)  [unwired: 1 in, 1 out]
            n1760 = local write "Position"(w3741) -> ()
            n1761 = property on="Position" class="Str"("Visible"=TRUE) -> ()  [unwired: 2 in, 2 out]
            n1762 = Bundle By Name(cluster=w3750, "RptUUT.Position"=w3741) -> (w3747:T73)
            n1763 = Unbundle By Name(w3746) -> ("Log"=w3744:refnum<class "Event Notification.lvclass">)
            n1764 = Format Into String(format string="UUT Position is %s" ("Message"), w3741) -> (resulting string=w3745:string)  [unwired: 2 in, 1 out]
            n1765 = call <vilib>:"Event Notification.Status Message.vi"("Log"=TRUE, "Level"=Event_Log.Log_Level."Verbose", "Message"=w3745, "Event Notification in"=w3744) -> ()  [unwired: 8 in]
          }
          frame "Set Variables" {
            # "SetVariable(Name,Value)"
            n1766 = Variant To Data(type=string[][] [], Variant=w3765) -> (data=w3753:string[][], error out=w3759:errorcluster)  [unwired: 1 in]
            n1767 = Unbundle By Name(w3763) -> ("SeqMgr"=w3762:refnum<class "SeqMgr.lvclass">)
            n1768 = local read "Variables"() -> (w3754:string[][])
            n1769 = call <vilib>:"SeqMgr.Variables - Add, Replace.vi"("Name, Value"=w3753, "SeqMgr in"=w3762) -> ("SeqMgr out"=w3761:refnum<class "SeqMgr.lvclass">)  [unwired: 8 in, 1 out]
            n1770 = Bundle By Name(cluster=w3763, "SeqMgr"=w3761) -> (w3757:T73)
            n1771 = call "TestExec.Add New 1D Items to 2D List, Overwrite if is existing.vi"("New Items"=w3753, "Item List"=w3754) -> ("Item List Out"=w3752:string[][])  [unwired: 9 in]
            n1772 = local write "Variables"(w3752) -> ()
            n1773 = Unbundle By Name(w3755) -> ("Log"=w3756:refnum<class "Event Notification.lvclass">)
            n1774 = for {
              tunnel: w3756 -> [w3768]
              tunnel: w3753 -> [w3770] mode=indexing
              n1775 = Index Array(array=w3770) -> (element #1=w3772:string, element #2=w3771:string)  [unwired: 2 in]
              n1776 = Format Into String(format string="Set Var, %s, %s", w3772, w3771) -> (resulting string=w3767:string)  [unwired: 2 in, 1 out]
              n1777 = call <vilib>:"Event Notification.Status Message.vi"("Log"=TRUE, "Level"=Event_Log.Log_Level."Debug0", "Message"=w3767, "Event Notification in"=w3768) -> ()  [unwired: 8 in]
            }
            n1778 = case shown="No Error" w3759 {
              selector: w3759 -> [_ w3779]
              tunnel: w3758 -> [_ w3776]
              tunnel: [_ w3774] -> w3760
              frame No Error {
              }
              frame Error {
                n1779 = Format Into String(format string="Invalid Data to task %s. Expected 1D string.", w3776) -> (resulting string=w3775:string)  [unwired: 2 in, 1 out]
                n1780 = call "Error.Set-Change Error Info.vi"("error in"=w3779, "Description"=w3775, "Cust Code(0 = no change)"=-5500 ("Code(0 = no change)")) -> ("error out"=w3774:errorcluster)  [unwired: 8 in]
              }
            }
          }
          frame "Sta Notify" {
            n1781 = Unbundle By Name(w3789) -> ("StaApp"=w3788:string, "StaNotify"=w3787:bool, "ResultState.State"=w3784:T1)
            n1782 = local read "Position"() -> (w3780:string)
            n1783 = property on="Sequence" class="Ring (strict)"() -> ("RingText.Text"=w3783:string, "Strings []"=w3782:string[])  [unwired: 2 in, 2 out]
            n1784 = local read "SN"() -> (w3781:string)
            n1785 = local read "Test State"() -> (w3785:enum32{"Idle", "Running", "Completed"})
            n1786 = property on="PLC" class="Bool (strict)"() -> ("Visible"=w3786:bool)  [unwired: 2 in, 2 out]
            n1787 = case shown="True" w3786 {
              tunnel: w3785 -> [_ w3792]
              tunnel: w3784 -> [_ w3791]
              frame False {
              }
              frame True {
                n1788 = case shown="Default" w3792 {
                  tunnel: w3791 -> [_ _ _ w3797]
                  frame Default {
                  }
                  frame "Idle" {
                    n1789 = call <vilib>:"Q.Enqueue Task.vi"("Q Name"="PLC", "Task Name"="TE Idle") -> ()  [unwired: 8 in, 2 out]
                  }
                  frame "Running" {
                    n1790 = call <vilib>:"Q.Enqueue Task.vi"("Q Name"="PLC", "Task Name"="TE Running") -> ()  [unwired: 8 in, 2 out]
                  }
                  frame "Completed" {
                    w3799 = "PLC" ("Q Name")
                    n1791 = case shown="\"Failing\", \"FAIL\", \"ERROR\"" w3797 {
                      tunnel: ["PASS" ("Task Name") "FAIL" ("Task Name")] -> w3801
                      frame "None", "PASS", Default {
                      }
                      frame "Failing", "FAIL", "ERROR" {
                      }
                    }
                    n1792 = To Variant(anything=w3801) -> (Variant=w3802:variant)
                    n1793 = call <vilib>:"Q.Enqueue Task.vi"("Data1"=w3802, "Q Name"=w3799, "Task Name"="TE Result") -> ("error out"=w3798:errorcluster)  [unwired: 7 in, 1 out]
                    n1794 = call <vilib>:"Q.Enqueue Task.vi"("Q Name"=w3799, "Error In"=w3798, "Task Name"="TE Complete") -> ()  [unwired: 7 in, 2 out]
                  }
                }
              }
            }
            n1795 = case shown="True" w3787 {
              tunnel: w3788 -> [_ w3814]
              tunnel: w3785 -> [_ w3813]
              tunnel: w3784 -> [_ w3812]
              tunnel: w3783 -> [_ w3809]
              tunnel: w3782 -> [_ w3808]
              tunnel: w3781 -> [_ w3807]
              tunnel: w3780 -> [_ w3806]
              frame False {
              }
              frame True {
                n1796 = Bundle By Name(cluster=T54 {"Test State"=enum."Idle", "Result"=enum."None", "Sequence"="", "Sequences"=[], "SN"="", "Position"=""} ("output cluster"), "Test State"=w3813, "Result"=w3812, "Sequence"=w3809, "Sequences"=w3808, "SN"=w3807, "Position"=w3806) -> (w3811:T54)
                n1797 = To Variant(anything=w3811) -> (Variant=w3815:variant)
                n1798 = call <vilib>:"Q.Enqueue Task.vi"("Data1"=w3815, "Q Name"=w3814, "Task Name"="TE State") -> ()  [unwired: 7 in, 2 out]
              }
            }
          }
          frame "Sta Set Config" {
            n1799 = Unbundle By Name(w3822) -> ("StaApp"=w3821:string)
            n1800 = Unbundle By Name(w3819) -> ("AppData"=w3818:refnum<class "Class.AppData.lvclass">)
            n1801 = call <vilib>:"ClassAppData.Get All.vi"("Class - App Data in"=w3818) -> ("Data Out"=w3817:variant)  [unwired: 8 in, 2 out]
            n1802 = call <vilib>:"Q.Enqueue Task.vi"("Data1"=w3817, "Q Name"=w3821, "Task Name"="Set Config") -> ()  [unwired: 7 in, 2 out]
          }
          frame "Sta Notify Set" {
            # "Sync with requestor"
            # "Turn ON or OFF test station app notifications to the station about the TE State\nThis is used when the station remotely interacts with TE."
            n1803 = Variant To Data(type=TRUE, Variant=w3829) -> (data=w3826:bool, error out=w3827:errorcluster)  [unwired: 1 in]
            n1804 = case shown="No Error" w3827 {
              tunnel: w3826 -> [w3833 _]
              tunnel: [w3833 _] -> w3825
              frame No Error {
              }
              frame Error {
              }
            }
            n1805 = call <vilib>:"Q.Enqueue Task.vi"("Task Name"="Sta Notify", "Q In"=w3824) -> ()  [unwired: 8 in, 2 out]
            n1806 = Bundle By Name(cluster=w3831, "StaNotify"=w3825) -> (w3830:T73)
          }
          frame "Sta Notify Ver" {
            n1807 = Variant To Data(type=0, Variant=w3839) -> (data=w3837:i32, error out=w3838:errorcluster)  [unwired: 1 in]
            n1808 = case shown="No Error" w3838 {
              tunnel: w3837 -> [w3845 _]
              tunnel: [w3845 _] -> w3834
              frame No Error {
              }
              frame Error {
              }
            }
            n1809 = case shown="1, Default" w3834 {
              tunnel: w3836 -> [_ w3844]
              frame 0 {
              }
              frame 1, Default {
                n1810 = call <vilib>:"Q.Enqueue Task.vi"("Task Name"="Sta Set Config", "Q In"=w3844) -> ()  [unwired: 8 in, 2 out]
              }
            }
            n1811 = Bundle By Name(cluster=w3841, "Lists.StaVer"=w3834) -> (w3840:T73)
          }
          frame "Sta Set TimeOut" {
            n1812 = Unbundle By Name(w3851) -> ("StaApp"=w3850:string, "TimeOut(s)"=w3846:dbl)
            n1813 = To Variant(anything=w3846) -> (Variant=w3847:variant)
            n1814 = call <vilib>:"Q.Enqueue Task.vi"("Top of Q"=TRUE, "Data1"=w3847, "Q Name"=w3850, "Task Name"="Set TimeOut") -> ()  [unwired: 6 in, 2 out]
          }
          frame "Sta Test Mode" {
            n1815 = Unbundle By Name(w3857) -> ("StaApp"=w3856:string)
            n1816 = property on="Mode" class="Ring (strict)"() -> ("RingText.Text"=w3853:string)  [unwired: 2 in, 2 out]
            n1817 = To Variant(anything=w3853) -> (Variant=w3854:variant)
            n1818 = call <vilib>:"Q.Enqueue Task.vi"("Data1"=w3854, "Q Name"=w3856, "Task Name"="Test Mode") -> ()  [unwired: 7 in, 2 out]
          }
          frame "Sta Test Reset" {
            n1819 = Unbundle By Name(w3861) -> ("StaApp"=w3860:string)
            n1820 = call <vilib>:"Q.Enqueue Task.vi"("Q Name"=w3860, "Task Name"="Test Reset") -> ()  [unwired: 8 in, 2 out]
          }
          frame "Sta Test Status" {
            n1821 = Unbundle By Name(w3868) -> ("StaApp"=w3867:string, "ResultState"=w3863:T63)
            n1822 = To Variant(anything=w3863) -> (Variant=w3864:variant)
            n1823 = call <vilib>:"Q.Enqueue Task.vi"("Top of Q"=TRUE, "Data1"=w3864, "Q Name"=w3867, "Task Name"="Test Status") -> ()  [unwired: 6 in, 2 out]
          }
          frame "StaCmd" {
            n1824 = Variant To Data(type=string[] [], Variant=w3878) -> (data=w3877:string[])  [unwired: 1 in, 1 out]
